vi "Read Read Only.vi"(8 "error in (no error)":errorcluster, 11 "Const_Current Time in":refnum<class "Const_Current Time.lvclass">) -> (0 "error out":errorcluster, 2 "Read Only":bool, 3 "Const_Current Time out":refnum<class "Const_Current Time.lvclass">)   [LabVIEW 2021, in "Const_Current Time.lvclass"]
uses:
  Const_Current Time.lvclass
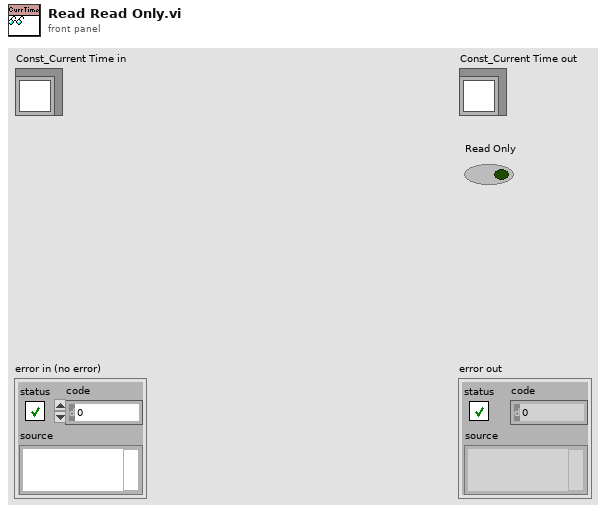
[diagram p1: front panel]
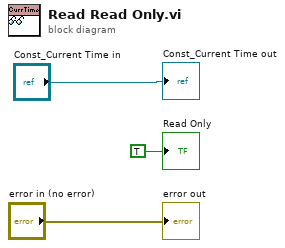
[diagram p0: block diagram]
diagram:
  "error out" <- "error in (no error)"
  "Const_Current Time out" <- "Const_Current Time in"
  "Read Only" <- TRUE ("Read Only")
